vi "Get_VIParamInformation.vi"(8 "error in (no error)":errorcluster, 10 "Compatibility":bool, 11 "path":path) -> (0 "error out":errorcluster, 3 "ExportAssemblyVIinfo out":T1)   [LabVIEW 2020]
uses:
  <vilib>/Utility/VariantDataType/VariantType.lvlib
  <vilib>/AppBuilder/AB_InteropAssembly_DistVI_Proto_Info.ctl
  <vilib>/AppBuilder/IOStatus.ctl
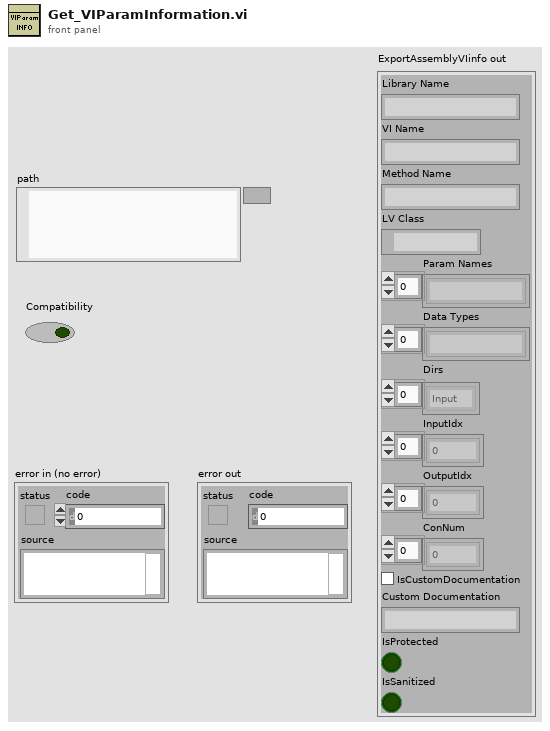
[diagram p1: front panel]
types:
  T1 = typedef "AB_InteropAssembly_DistVI_Proto_Info.ctl" = cluster{"Library Name":string, "VI Name":string, "Method Name":string, "LV Class":path, "Param Names":string[], "Data Types":string[], "Dirs":T2[], "InputIdx":i32[], "OutputIdx":i32[], "ConNum":i8[], "IsCustomDocumentation":bool, "Custom Documentation":string, "IsProtected":bool, "IsSanitized":bool}
  T2 = typedef "IOStatus.ctl" = enum16{"Input", "Output", "Input/Output", "InputDeleted", "OutputDeleted", "IODeleted", "ErrorClusterIn", "ErrorClusterOut"}
  T3 = typedef "VariantType.lvlib/VIInfo.ctl" = cluster{"Data1":i16, "Data2":i16, "Flags":u32[], "Modification Date":timestamp, "Asynchronous":bool, "NonFunctional":bool, "Subroutine":bool, "SubSystem":bool}
  T4 = typedef "LVRectTypeDef.ctl" = cluster{"Left":i16, "Top":i16, "Right":i16, "Bottom":i16}
  T5 = typedef "VariantType.lvlib/Type.ctl" = enum8{"Invalid Type", "Void", "I8", "I16", "I32", "I64", "U8", "U16", "U32", "U64", "Single Float", "Double Float", "Extended Float", "Single Complex", "Double Complex", "Extended Complex", "Enum U8", "Enum U16", "Enum U32", "Enum U64", "Single Float With Unit", "Double Float With Unit", "Extended Float With Unit", "Single Complex with Unit", "Double Complex with Unit", "Extended Complex with Unit", "Boolean", "String", "Path", "Picture", "Tag", "Array", "Cluster", "Variant", "LV Variant", "Waveform", "Timestamp", "Digital Waveform", "Digital Data", "ExpressData", "Refnum", "External Data", "VI", "Poly VI", "LabVIEW Class Instance", "Fixed Point"}
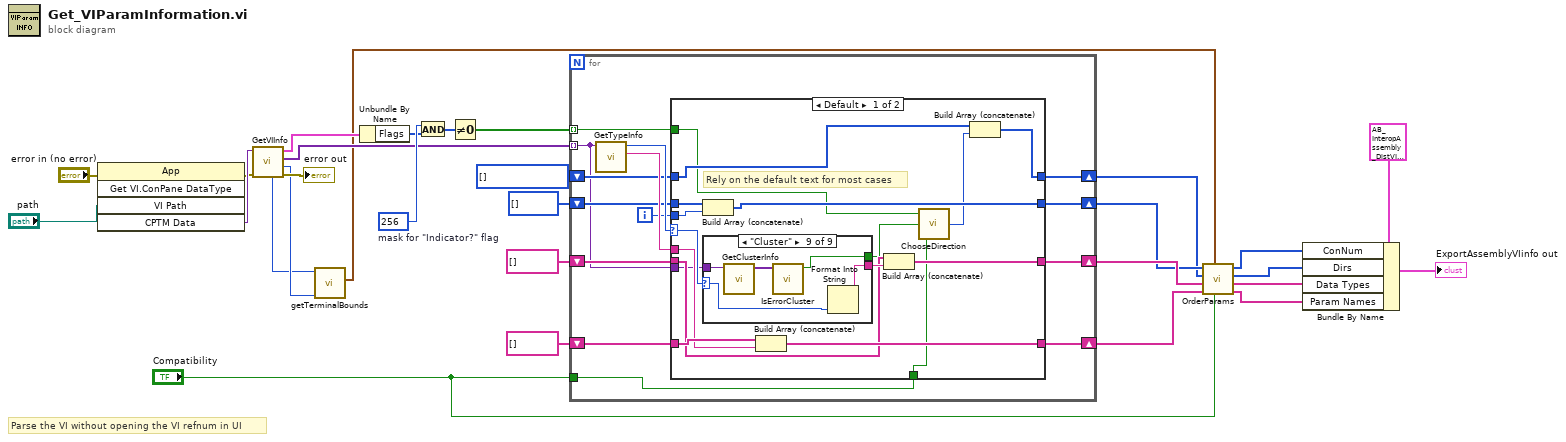
[diagram p0: block diagram]
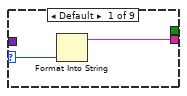
[diagram p2: hidden frame]
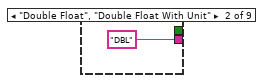
[diagram p3: hidden frame]
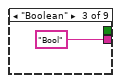
[diagram p4: hidden frame]
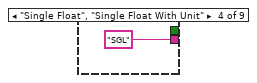
[diagram p5: hidden frame]
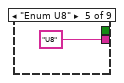
[diagram p6: hidden frame]
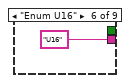
[diagram p7: hidden frame]
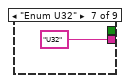
[diagram p8: hidden frame]
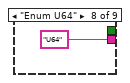
[diagram p9: hidden frame]
diagram:
  w26 = T2[] [] items=["Input", "Output", "Input/Output", "InputDeleted", "OutputDeleted", "IODeleted", "ErrorClusterIn", "ErrorClusterOut"]
  w22 = i16 256  # mask for "Indicator?" flag
  # "Parse the VI without opening the VI refnum in UI"
  n1 = invoke class="App" method="Get VI.ConPane DataType"(error in="error in (no error)", "VI Path"="path") -> (error out=w16:errorcluster, "CPTM Data"=w17:variant)  [unwired: 3 in, 3 out]
  n2 = call <vilib>:"GetVIInfo.vi"("error in (no error)"=w16, "Variant"=w17) -> ("error out"=→"error out":errorcluster, "permutation"=w12:i16, "VI Terminal Types"=w20:variant[], "VI Info"=w25:T3, "pattern"=w11:i16)  [unwired: 5 out]
  n3 = call <vilib>:"getTerminalBounds.VI"("Permutation"=w12, "Pattern"=w11) -> ("Terminal Bounds[]"=w2:T4[])  [unwired: 9 in]
  n4 = Unbundle By Name(w25) -> ("Flags"=w21:u32[])
  n5 = And(x=w22, y=w21) -> (x .and. y?=w23:u32[])
  n6 = Not Equal To 0?(x=w23) -> (x != 0?=w24:bool[])
  n7 = for {
    tunnel: w20 -> [w31] mode=indexing
    tunnel: w24 -> [w41] mode=indexing
    shift-right: [w40] -> w3
    shift-left: w26 -> [w39]
    shift-right: [w37] -> w6
    shift-left: string[] [] -> [w36]
    shift-right: [w35] -> w5
    shift-left: string[] [] -> [w34]
    shift-right: [w32] -> w4
    shift-left: i8[] [] -> [w33]
    tunnel: "Compatibility" -> [w30]
    i -> [w38]
    n8 = call <vilib>:"GetTypeInfo.vi"("Variant"=w31) -> ("Name"=w42:string, "Type Enum"=w43:T5)  [unwired: 1 in, 8 out]
    n9 = case shown="Default" w43 {
      selector: w43 -> [w56 _]
      tunnel: w42 -> [w51 _]
      tunnel: w41 -> [w46 _]
      tunnel: [w60 w78] -> w40
      tunnel: w39 -> [w53 w78]
      tunnel: [w59 w75] -> w32
      tunnel: w38 -> [w54 _]
      tunnel: w33 -> [w55 w75]
      tunnel: [w58 w77] -> w37
      tunnel: w36 -> [w49 w77]
      tunnel: [w57 w76] -> w35
      tunnel: w34 -> [w52 w76]
      tunnel: w31 -> [w48 _]
      tunnel: w30 -> [w44 _]
      frame Default {
        # "Rely on the default text for most cases"
        n10 = Build Array (concatenate)(w55, w54) -> (w59:i32[])
        n11 = case shown="\"Cluster\"" w56 {
          selector: w56 -> [w62 _ _ _ _ _ _ _ w72]
          tunnel: [w61 "DBL" ("Boolean Text") "Bool" ("Boolean Text") "SGL" ("Boolean Text") "U8" ("Boolean Text") "U16" ("Boolean Text") "U32" ("Boolean Text") "U64" ("Boolean Text") w71] -> w50
          tunnel: w48 -> [_ _ _ _ _ _ _ _ w73]
          tunnel: [_ _ _ _ _ _ _ _ w70] -> w47
          frame Default {
            n12 = Format Into String(w62) -> (resulting string=w61:string)  [unwired: 3 in, 1 out]
          }
          frame "Double Float", "Double Float With Unit" {
          }
          frame "Boolean" {
          }
          frame "Single Float", "Single Float With Unit" {
          }
          frame "Enum U8" {
          }
          frame "Enum U16" {
          }
          frame "Enum U32" {
          }
          frame "Enum U64" {
          }
          frame "Cluster" {
            n13 = call <vilib>:"GetClusterInfo.vi"("Variant"=w73) -> ("Cluster Elements"=w74:variant[])  [unwired: 9 in, 1 out]
            n14 = call <vilib>:"IsErrorCluster.vi"("Cluster Elements"=w74) -> ("Boolean"=w70:bool)  [unwired: 8 in]
            n15 = Format Into String(w72) -> (resulting string=w71:string)  [unwired: 3 in, 1 out]
          }
        }
        n16 = Build Array (concatenate)(w52, w51) -> (w57:string[])
        n17 = Build Array (concatenate)(w49, w50) -> (w58:string[])
        n18 = call <vilib>:"ChooseDirection.vi"("UseLV2011Compatibility"=w44, "IsErrorCluster"=w47, "ISOutput"=w46) -> ("Dir 2"=w45:T2)
        n19 = Build Array (concatenate)(w53, w45) -> (w60:T2[])
      }
      frame "Void" {
      }
    }
  }
  n20 = call <vilib>:"OrderParams.vi"("UseLV2011Compatability"="Compatibility", "Terminal Bounds[]"=w2, "Param Names"=w5, "Data types"=w6, "Dirs"=w3, "Connum"=w4) -> ("Param Names out"=w7:string[], "Data types  out"=w8:string[], "Dirs Out"=w9:T2[], "Connum out"=w10:i32[])  [unwired: 2 in]
  n21 = Bundle By Name(cluster=T1 {"Library Name"="", "VI Name"="", "Method Name"="", "LV Class"=path "", "Param Names"=[], "Data Types"=[], "Dirs"=[], "InputIdx"=[], "OutputIdx"=[], "ConNum"=[], "IsCustomDocumentation"=FALSE, "Custom Documentation"="", "IsProtected"=FALSE, "IsSanitized"=FALSE} ("ExportAssemblyVIinfo out"), "ConNum"=w10, "Dirs"=w9, "Data Types"=w8, "Param Names"=w7) -> (→"ExportAssemblyVIinfo out":T1)
